vi "Read.vi"(7 "I2C Channel (0)":u8, 8 "Error In":errorcluster, 9 "Resolution (dps)":enum16{"2000", "500", "250"}(ring), 10 "I2C Slave Address":enum8{"0x68", "0x69"}(ring)=enum."0x69", 11 "LINX Resource":T1) -> (0 "Error Out":errorcluster, 2 "Rotation(dps)":cluster{"X":i16, "Y":i16, "Z":i16}, 3 "LINX Resource":T1)   [LabVIEW 2014, in "LMH-LINX.lvlib" / "PmodGYRO.lvlib"]
doc: "Read X, Y and Z axis rotation data from the PmodGYRO in degrees per second (dps)."
uses:
  <vilib>/MakerHub/LINX/Public/Sensors/Pmods/GYRO/PmodGYRO.lvlib
  <vilib>/MakerHub/LINX/Private/Type Defs/LINX Ref.ctl
  <vilib>/MakerHub/LINX/Private/Type Defs/Platform.ctl
  <vilib>/MakerHub/LINX/Private/Type Defs/Interface.ctl
  <vilib>/MakerHub/LINX/Private/Device/Type Defs/LINX Device Config.ctl
  <vilib>/MakerHub/LINX/Private/Device/Type Defs/TCP Config.ctl
  <vilib>/MakerHub/LINX/Private/Device/Type Defs/Channels.ctl
  <vilib>/MakerHub/LINX/Private/Local IO/LinxI2cWrite.vi
  <vilib>/MakerHub/LINX/Public/Utilities/Check Channel.vi
  <vilib>/MakerHub/LINX/Private/Utilties/Generate Error.vi
  <vilib>/MakerHub/LINX/LMH-LINX.lvlib
  <vilib>/MakerHub/Toolbox/LMH-Toolbox.lvlib
  <vilib>/MakerHub/LINX/Private/Device/Device.lvlib
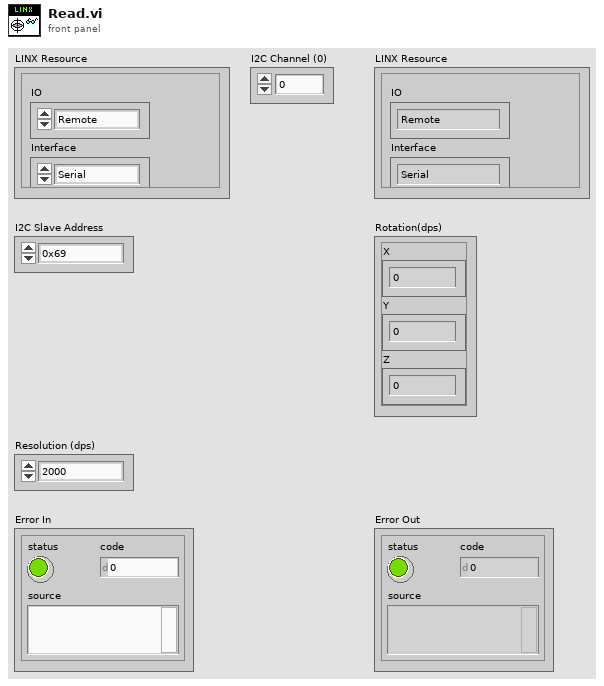
[diagram p1: front panel]
types:
  T1 = typedef "LMH-LINX.lvlib/LINX Ref.ctl" = cluster{"IO":T2, "Interface":T3, "LINX Device Config":T4}
  T2 = typedef "LMH-LINX.lvlib/Platform.ctl" = enum16{"Remote", "Local"}
  T3 = typedef "LMH-LINX.lvlib/Interface.ctl" = enum16{"Serial", "TCP"}
  T4 = typedef "LMH-LINX.lvlib/Device.lvlib/LINX Device Config.ctl" = cluster{"Interface":T3, "COM Port":refnum<visa-resource-name>, "TCP Configuration":T5, "Device Family":u8, "Device ID":u8, "Device Name":string, "TCP Ref":refnum<k5>, "Channels":T6}
  T5 = typedef "LMH-LINX.lvlib/Device.lvlib/TCP Config.ctl" = cluster{"IP Address":string, "Port":u16}
  T6 = typedef "LMH-LINX.lvlib/Channels.ctl" = cluster{"DI":u8[], "DO":u8[], "AI":u8[], "AO":u8[], "PWM":u8[], "QE":u8[], "UART":u8[], "I2C 2":u8[], "SPI":u8[], "CAN":u8[], "Servo":u8[], "AI Ref (V)":dbl, "AI Resolution (Bits)":u8, "AO Ref (V)":dbl, "AO Resolution (Bits)":u8}
  T7 = cluster{"Decimal I16":i16, "Decimal I16":i16, "Decimal I16":i16}
  T8 = cluster{"Decimal I16":dbl, "Decimal I16":dbl, "Decimal I16":dbl}
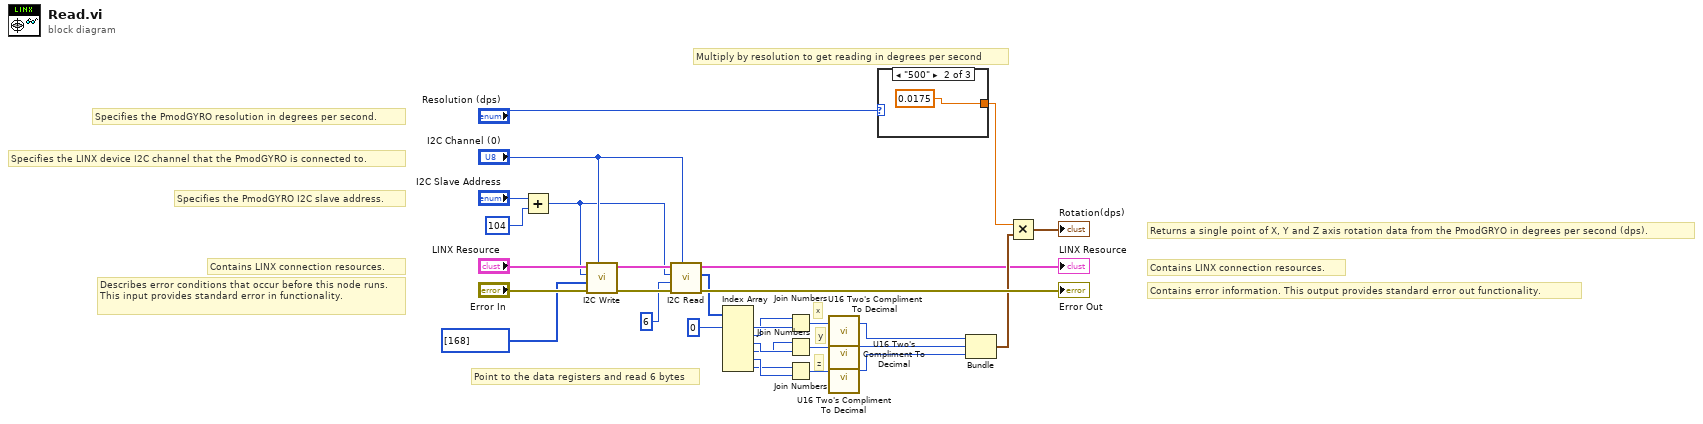
[diagram p0: block diagram]
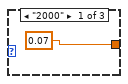
[diagram p2: hidden frame]
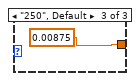
[diagram p3: hidden frame]
diagram:
  # "Specifies the PmodGYRO resolution in degrees per second."
  # "Specifies the PmodGYRO I2C slave address."
  # "Specifies the LINX device I2C channel that the PmodGYRO is connected to."
  # "Returns a single point of X, Y and Z axis rotation data from the PmodGRYO in degrees per second (dps)."
  # "Contains LINX connection resources."
  # "Contains error information. This output provides standard error out functionality."
  # "Contains LINX connection resources."
  # "Describes error conditions that occur before this node runs. This input provides standard error in functionality."
  # "Multiply by resolution to get reading in degrees per second"
  # "Point to the data registers and read 6 bytes"
  # "z"
  # "y"
  # "x"
  n1 = Add(x="I2C Slave Address", y=u8 104) -> (x+y=w7:u8)
  n2 = call <vilib>:"I2C Write.vi"("I2C Channel"="I2C Channel (0)", "Error In"="Error In", "Data"=u8[] [168], "I2C Slave Address (0)"=w7, "LINX Resource"="LINX Resource") -> ("Error Out"=w13:errorcluster, "LINX Resource"=w15:T1)  [unwired: 5 in]
  n3 = call <vilib>:"I2C Read.vi"("I2C Channel"="I2C Channel (0)", "Error In"=w13, "Bytes To Read"=u8 6, "I2C Slave Address (0)"=w7, "LINX Resource"=w15) -> ("Error Out"=→"Error Out":errorcluster, "Data"=w17:u8[], "LINX Resource"=→"LINX Resource":T1)  [unwired: 4 in]
  n4 = Index Array(array=w17, index #1=0 ("index")) -> (element #1=w6:u8, element #2=w5:u8, element #3=w4:u8, element #4=w3:u8, element #5=w2:u8, element #6=w1:u8)  [unwired: 5 in]
  n5 = Join Numbers(hi=w5, lo=w6) -> ((hi.lo)=w20:u16)
  n6 = Join Numbers(hi=w3, lo=w4) -> ((hi.lo)=w22:u16)
  n7 = Join Numbers(hi=w1, lo=w2) -> ((hi.lo)=w21:u16)
  n8 = call <vilib>:"U16 Two's Compliment To Decimal.vi"("Two's Compliment U16"=w20) -> ("Decimal I16"=w23:i16)  [unwired: 2 in]
  n9 = call <vilib>:"U16 Two's Compliment To Decimal.vi"("Two's Compliment U16"=w22) -> ("Decimal I16"=w24:i16)  [unwired: 2 in]
  n10 = call <vilib>:"U16 Two's Compliment To Decimal.vi"("Two's Compliment U16"=w21) -> ("Decimal I16"=w25:i16)  [unwired: 2 in]
  n11 = case shown="\"500\"" "Resolution (dps)" {
    tunnel: [0.07 0.0175 0.00875] -> w27
    frame "2000" {
    }
    frame "500" {
    }
    frame "250", Default {
    }
  }
  n12 = Bundle("Decimal I16"=w23, "Decimal I16"=w24, "Decimal I16"=w25) -> (w26:T7)  [unwired: 1 in]
  n13 = Multiply(x=w27, y=w26) -> (x*y=→"Rotation(dps)":T8)
